vi "Kinect.vi"() -> ()   [LabVIEW 2017]
uses:
  <vilib>/MakerHub/KinectOne/Private/kinectRead [DepthFrame].vi
  <vilib>/MakerHub/KinectOne/Private/Initialize Image [Depth].vi
  <vilib>/MakerHub/KinectOne/KinectOne.lvlib
panel:
  out "Body Index Image":T1(plugin-control)
  in  "stop":bool
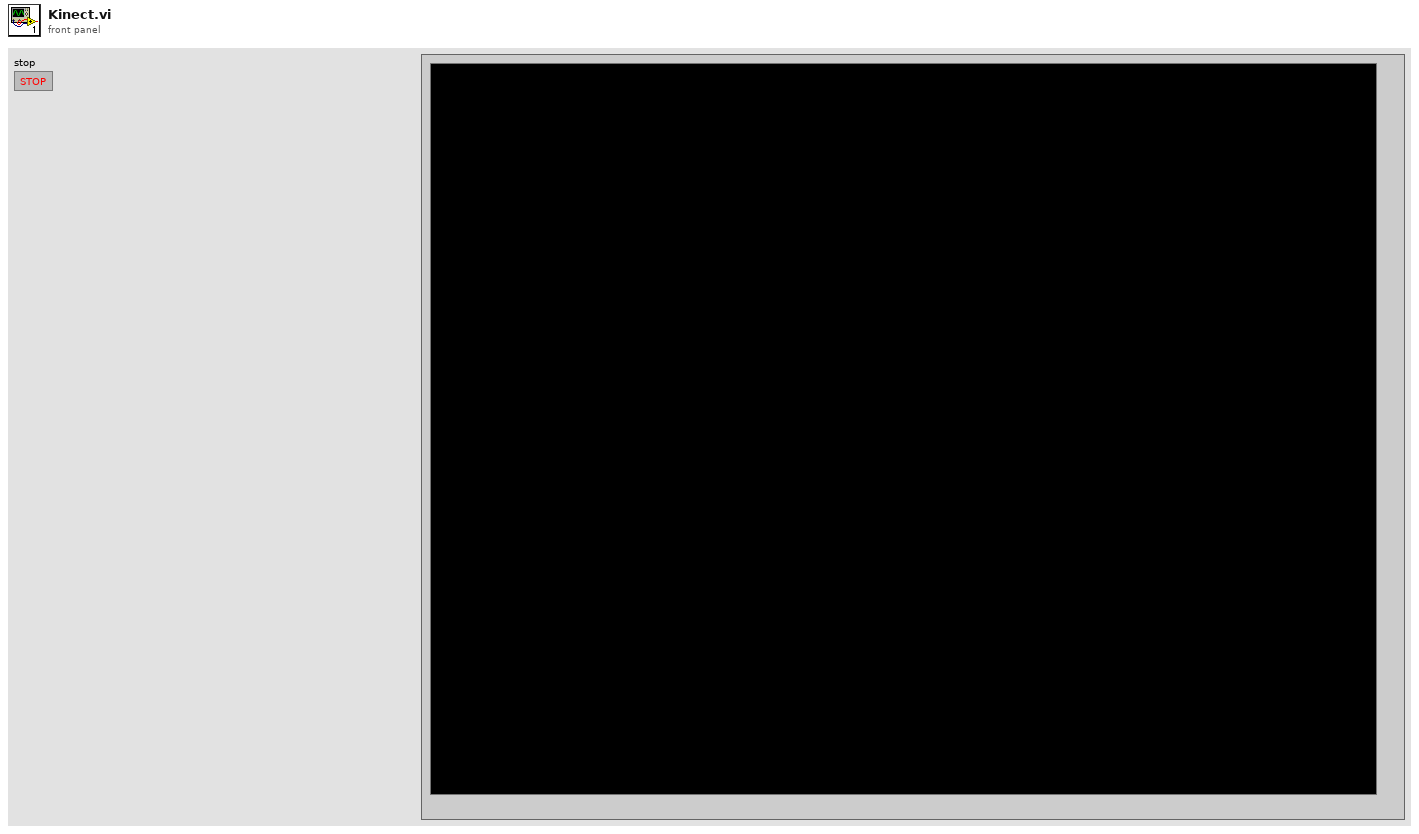
[diagram p1: front panel]
types:
  T1 = typedef "IMAQ Image.ctl" = refnum<image>
  T2 = typedef "KinectOne.lvlib/KinectSensor References.ctl" = cluster{"KinectSensor":refnum<k24>, "MultiSourceFrameReader":refnum<k24>, "BodyFrameDataInterface":refnum<k24>}
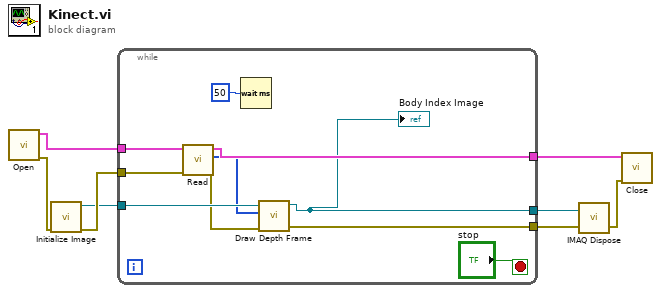
[diagram p0: block diagram]
diagram:
  n1 = call <vilib>:"Open.vi"() -> ("Error Out"=w8:errorcluster, "KinectSensor References out"=w7:T2)  [unwired: 10 in]
  n2 = call-poly <vilib>:"Initialize Image.vi"("Error In"=w8) -> ("Error Out"=w5:errorcluster, "Depth Image"=w4:T1)  [unwired: 9 in]
  n3 = while {
    tunnel: w7 -> [w18]
    tunnel: [w17] -> w6
    tunnel: w5 -> [w16]
    tunnel: w4 -> [w15]
    tunnel: [w12] -> w2
    tunnel: [w10] -> w1
    stop <- "stop" stop-if-true
    n4 = call-poly <vilib>:"Read.vi"("Error In"=w16, "KinectSensor References in"=w18) -> ("Error Out"=w13:errorcluster, "frameData"=w14:u16[], "KinectSensor References out"=w17:T2)  [unwired: 7 in]
    n5 = Wait (ms)(milliseconds to wait=u32 50) -> ()  [unwired: 1 out]
    n6 = call <vilib>:"Draw Depth Frame.vi"("Error In"=w13, "U16 Array"=w14, "Image"=w15) -> ("Error Out"=w12:errorcluster, "Image Out"=w10:T1)  [unwired: 7 in]
    "Body Index Image" <- w10
  }
  n7 = call "IMAQ Dispose"("Image"=w1, "error in (no error)"=w2) -> ("error out"=w3:errorcluster)  [unwired: 4 in]
  n8 = call <vilib>:"Close.vi"("Error In"=w3, "KinectSensor References"=w6) -> ()  [unwired: 9 in, 1 out]
